vi "反转判断1.vi"(6 "重置？":bool, 8 "error in (no error)":errorcluster caption="错误输入（无错误）", 9 "反转判断条件1":T1, 10 "传感器数据":dbl[](array[numeric]), 11 "Message Queues":T2 caption="消息队列") -> (0 "error out":errorcluster caption="错误输出", 2 "反转":bool)   [LabVIEW 2015, in "Motor Control.lvlib"]
uses:
  Motor Control.lvlib
  support/Message Queue/All Message Queues.ctl
  support/Message Queue/Message Cluster.ctl
  support/Message Queue/Enqueue Message (Single).vi
  support/Message Queue/Message Queue.lvlib
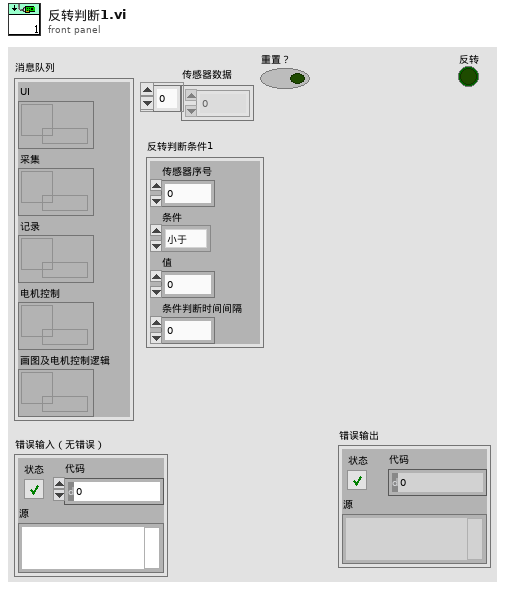
[diagram p1: front panel]
types:
  T1 = typedef "Motor Control.lvlib/反转判断条件1.ctl" = cluster{"传感器序号":i32, "条件":enum16{"小于", "大于", "等于"}, "值":dbl, "条件判断时间间隔":i32}
  T2 = typedef "Message Queue.lvlib/All Message Queues.ctl" = cluster{"UI":refnum<queue>, "Acquisition":refnum<queue>, "Logging":refnum<queue>, "MotorCtrl":refnum<queue>, "plot logic":refnum<queue>}
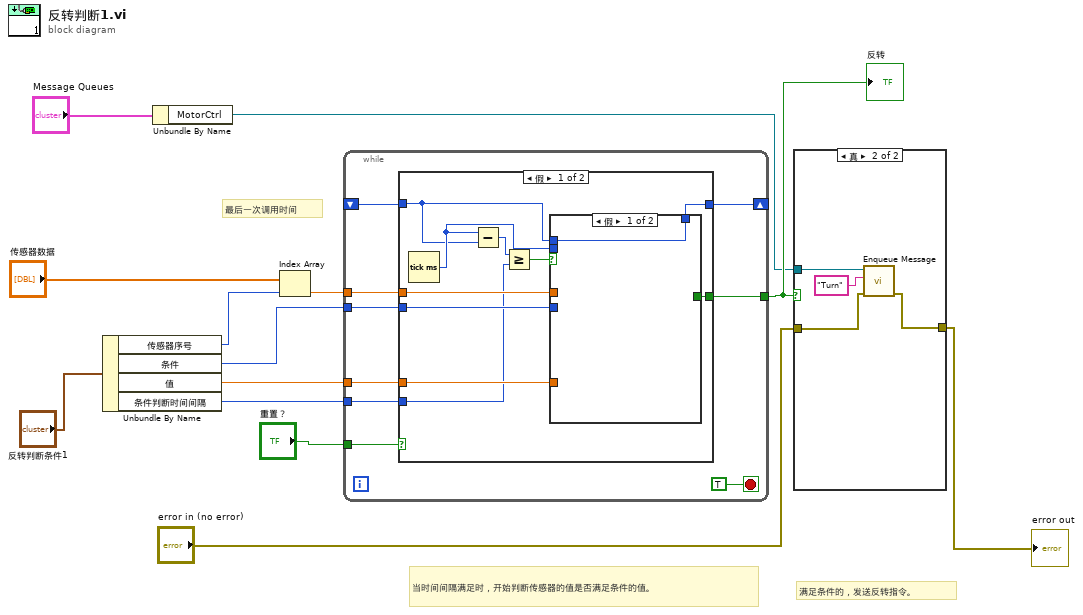
[diagram p0: block diagram]
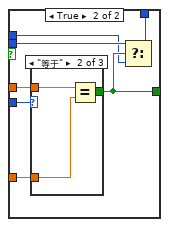
[diagram p3: hidden frame]
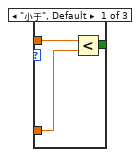
[diagram p4: hidden frame]
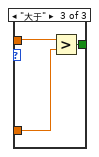
[diagram p5: hidden frame]
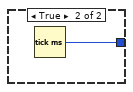
[diagram p6: hidden frame]
diagram:
  # "满足条件的，发送反转指令。"
  # "当时间间隔满足时，开始判断传感器的值是否满足条件的值。"
  # "最后一次调用时间"
  n1 = Unbundle By Name("反转判断条件1") -> ("传感器序号"=w10:i32, "条件"=w9:enum16{"小于", "大于", "等于"}, "值"=w7:dbl, "条件判断时间间隔"=w6:i32)
  n2 = Unbundle By Name("Message Queues") -> ("MotorCtrl"=w4:refnum<queue>)
  n3 = Index Array(array="传感器数据", index=w10) -> (element=w8:dbl)
  n4 = while {
    tunnel: w9 -> [w22]
    tunnel: w8 -> [w21]
    tunnel: w7 -> [w20]
    shift-right: [w19] -> _
    shift-left: _ -> [w18]
    tunnel: w6 -> [w17]
    tunnel: [w16] -> w5
    tunnel: "重置？" -> [w14]
    stop <- TRUE stop-if-true
    n5 = case shown="假" w14 {
      tunnel: w22 -> [w32 _]
      tunnel: w21 -> [w31 _]
      tunnel: w20 -> [w30 _]
      tunnel: [w23 w50] -> w19
      tunnel: w18 -> [w24 _]
      tunnel: w17 -> [w28 _]
      tunnel: [w26 _] -> w16
      frame False {
        n6 = Tick Count (ms)() -> (millisecond timer value=w25:u32)
        n7 = Subtract(x=w25, y=w24) -> (x-y=w29:u32)
        n8 = Greater Or Equal?(x=w29, y=w28) -> (x >= y?=w27:bool)
        n9 = case shown="假" w27 {
          tunnel: w32 -> [_ w40]
          tunnel: w31 -> [_ w39]
          tunnel: w30 -> [_ w38]
          tunnel: [_ w37] -> w26
          tunnel: w25 -> [_ w36]
          tunnel: w24 -> [w33 w35]
          tunnel: [w33 w34] -> w23
          frame False {
          }
          frame True {
            n10 = case shown="\"等于\"" w40 {
              tunnel: w39 -> [w43 w46 w49]
              tunnel: w38 -> [w42 w45 w48]
              tunnel: [w41 w44 w47] -> w37
              frame "小于", Default {
                n11 = Less?(x=w43, y=w42) -> (x < y?=w41:bool)
              }
              frame "等于" {
                n12 = Equal?(x=w46, y=w45) -> (x = y?=w44:bool)
              }
              frame "大于" {
                n13 = Greater?(x=w49, y=w48) -> (0:w47:bool)
              }
            }
            n14 = Select(t=w36, s=w37, f=w35) -> (s? t:f=w34:u32)
          }
        }
      }
      frame True {
        n15 = Tick Count (ms)() -> (millisecond timer value=w50:u32)
      }
    }
  }
  "反转" <- w5
  n16 = case shown="真" w5 {
    tunnel: w4 -> [_ w55]
    tunnel: "error in (no error)" -> [w51 w54]
    tunnel: [w51 w53] -> w2
    frame False {
    }
    frame True {
      n17 = call-poly "Enqueue Message.vi"("error in (no error)"=w54, "Message"="Turn", "Message Queue"=w55) -> ("error out"=w53:errorcluster)  [unwired: 7 in, 1 out]
    }
  }
  "error out" <- w2
